vi "gfitsio-check-col-for-read.vi"(4 "expected dimensionality":enum16{"scalar", "array"}(ring), 6 "row":i32, 7 "column":string, 8 "error in (no error)":errorcluster, 11 "gfits refnum":T1) -> (0 "error out":errorcluster, 2 "nelements":i32, 3 "dup gfits refnum":T1)   [LabVIEW 2011, in "gfitsio.lvlib"]
uses:
  gfitsio.lvlib
  gfitsio-refnum.ctl
  gfitsio-error-codes.ctl
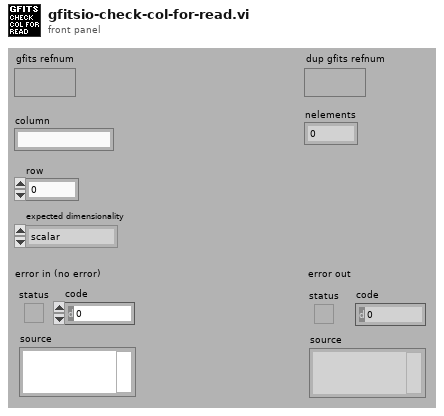
[diagram p1: front panel]
types:
  T1 = typedef "gfitsio.lvlib/gfitsio-refnum.ctl" = refnum<k1>
  T2 = typedef "gfitsio.lvlib/gfitsio-error-codes.ctl" = i32
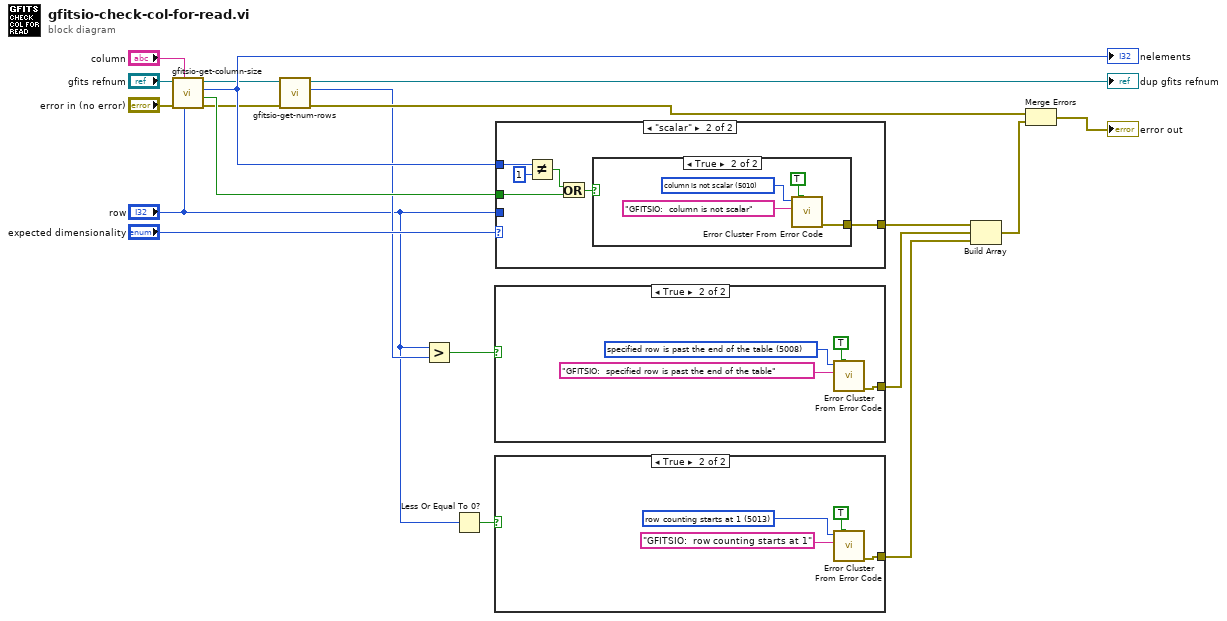
[diagram p0: block diagram]
diagram:
  n1 = call "gfitsio-get-column-size.vi"("row"="row", "column"="column", "error in (no error)"="error in (no error)", "gfits refnum"="gfits refnum") -> ("error out"=w12:errorcluster, "variable length?"=w19:bool, "nelements"=w15:i32, "dup gfits refnum"=w11:T1)  [unwired: 4 in]
  "nelements" <- w15
  n2 = call "gfitsio-get-num-rows.vi"("error in (no error)"=w12, "gfits refnum"=w11) -> ("error out"=w10:errorcluster, "number of rows"=w8:i32, "dup gfits refnum"=→"dup gfits refnum":T1)  [unwired: 7 in]
  n3 = Greater?(x="row", y=w8) -> (0:w7:bool)
  n4 = Less Or Equal To 0?(x="row") -> (x <= 0?=w3:bool)
  n5 = case shown="True" w7 {
    tunnel: [_ w22] -> w4
    frame False {
    }
    frame True {
      w20 = T2 5008 items=["no error"=0, "dimensionality conflict"=5001, "fpixel out of image bounds"=5002, "lpixel out of image bounds"=5003, "increment size larger than image"=5004, "increment must be greater than zero"=5005, "fpixel must specify lower left corner"=5006, "named HDU not found"=5007, "specified row is past the end of the table"=5008, "wrong number of elements for column"=5009, "column is not scalar"=5010, "duplicate HDU name"=5011, "invalid table type"=5012] ("error code (0)")
      n6 = call <vilib>:"Error Cluster From Error Code.vi"("show call chain? (False)"=TRUE, "error message (\"\")"="GFITSIO:  specified row is past the end of the table" ("error message (\"\")"), "error code (0)"=w20) -> ("error out"=w22:errorcluster)  [unwired: 6 in]
    }
  }
  n7 = case shown="True" w3 {
    tunnel: [_ w26] -> w1
    frame False {
    }
    frame True {
      w24 = T2 5013 items=["no error"=0, "dimensionality conflict"=5001, "fpixel out of image bounds"=5002, "lpixel out of image bounds"=5003, "increment size larger than image"=5004, "increment must be greater than zero"=5005, "fpixel must specify lower left corner"=5006, "named HDU not found"=5007, "specified row is past the end of the table"=5008, "wrong number of elements for column"=5009, "column is not scalar"=5010, "duplicate HDU name"=5011, "invalid table type"=5012, "row counting starts at 1"=5013] ("Ring")
      n8 = call <vilib>:"Error Cluster From Error Code.vi"("show call chain? (False)"=TRUE, "error message (\"\")"="GFITSIO:  row counting starts at 1" ("error message (\"\")"), "error code (0)"=w24) -> ("error out"=w26:errorcluster)  [unwired: 6 in]
    }
  }
  n9 = case shown="\"scalar\"" "expected dimensionality" {
    tunnel: [_ w28] -> w6
    tunnel: w15 -> [_ w29]
    tunnel: w19 -> [_ w31]
    tunnel: "row" -> [_ _]
    frame "array" {
    }
    frame "scalar" {
      n10 = Not Equal?(x=w29, y=1) -> (x != y?=w32:bool)
      n11 = Or(x=w32, y=w31) -> (x .or. y?=w30:bool)
      n12 = case shown="True" w30 {
        tunnel: [_ w35] -> w28
        frame False {
        }
        frame True {
          w36 = T2 5010 items=["no error"=0, "dimensionality conflict"=5001, "fpixel out of image bounds"=5002, "lpixel out of image bounds"=5003, "increment size larger than image"=5004, "increment must be greater than zero"=5005, "fpixel must specify lower left corner"=5006, "named HDU not found"=5007, "specified row is past the end of the table"=5008, "wrong number of elements for column"=5009, "column is not scalar"=5010, "duplicate HDU name"=5011, "invalid table type"=5012] ("error code (0)")
          n13 = call <vilib>:"Error Cluster From Error Code.vi"("show call chain? (False)"=TRUE, "error message (\"\")"="GFITSIO:  column is not scalar" ("error message (\"\")"), "error code (0)"=w36) -> ("error out"=w35:errorcluster)  [unwired: 6 in]
        }
      }
    }
  }
  n14 = Build Array(w6, w4, w1) -> (w5:errorcluster[])
  n15 = Merge Errors(w10, w5) -> (→"error out":errorcluster)
